vi "Funzioni stringhe.vi"() -> ()   [LabVIEW 2012]
panel:
  out "reversed":string
  out "first char last":string
  out "string array all'indice":string
  out "selection":bool
  out "match":string
  out "match + rest of string":string
  out "substring before match":string
  out "appended array":dbl[][](array[numeric])
  out "array":dbl[][](array[numeric])
  out "spreadsheet string":string
  out "number of replacements":i32
  out "result string dopo search e replace":string
  out "replaced substring":string
  out "result string dopo replace":string
  in  "Substringa":string="Pappappero"
  out "substring":string
  out "concatenated string":string
  out "length":i32
  in  "Stringa iniziale":string="Si sta come d'autunno sugli alberi le foglie."
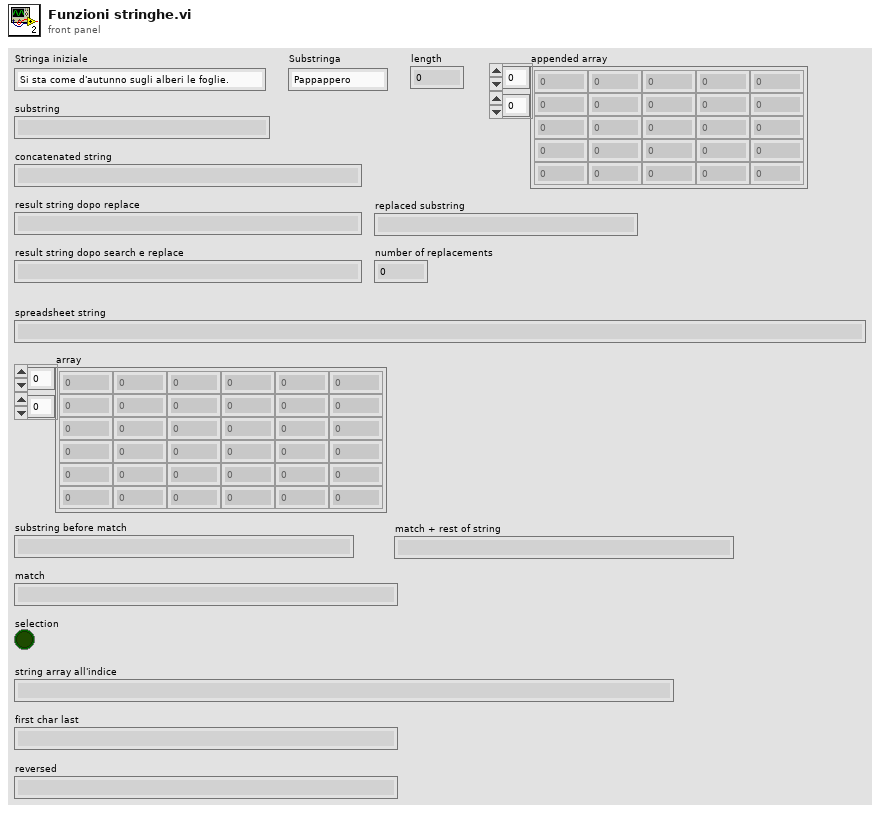
[diagram p1: front panel]
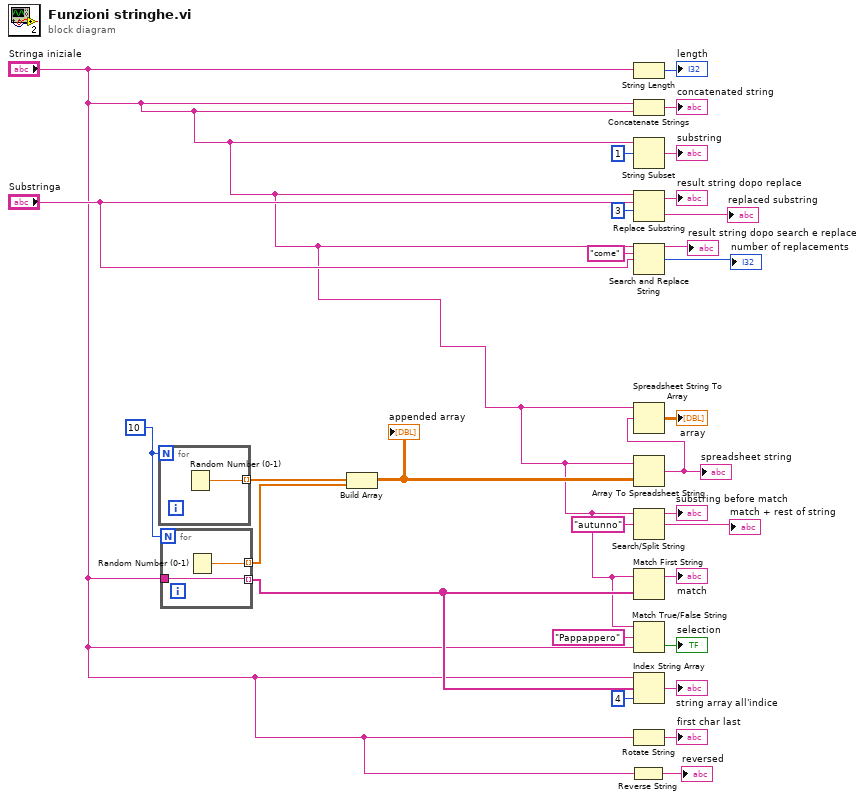
[diagram p0: block diagram]
diagram:
  w16 = 10
  n1 = for {
    N: w16 -> [_]
    tunnel: [w30] -> w17 mode=indexing
    n2 = Random Number (0-1)() -> (number: 0 to 1=w30:dbl)
  }
  n3 = for {
    N: w16 -> [_]
    tunnel: [w32] -> w18 mode=indexing
    tunnel: [w31] -> w8 mode=indexing
    tunnel: "Stringa iniziale" -> [w31]
    n4 = Random Number (0-1)() -> (number: 0 to 1=w32:dbl)
  }
  n5 = Build Array(w17, w18) -> (w15:dbl[][])
  "appended array" <- w15
  n6 = Reverse String(1:"Stringa iniziale") -> (0:→"reversed":string)
  n7 = String Length(string="Stringa iniziale") -> (length=→"length":i32)
  n8 = Concatenate Strings("Stringa iniziale", "Stringa iniziale") -> (→"concatenated string":string)
  n9 = String Subset(string="Stringa iniziale", offset (0)=1) -> (substring=→"substring":string)  [unwired: 1 in]
  n10 = Replace Substring(3:3 ("offset (0)"), 4:"Substringa", 5:"Stringa iniziale") -> (0:→"replaced substring":string, 1:→"result string dopo replace":string)  [unwired: 1 in]
  n11 = Search and Replace String(input string="Stringa iniziale", search string="come", replace string="Substringa") -> (result string=→"result string dopo search e replace":string, number of replacements=→"number of replacements":i32)  [unwired: 5 in, 2 out]
  n12 = Array To Spreadsheet String(array=w15, 3:"Stringa iniziale") -> (spreadsheet string=w14:string)  [unwired: 1 in]
  "spreadsheet string" <- w14
  n13 = Spreadsheet String To Array(format string="Stringa iniziale", spreadsheet string=w14) -> (array=→"array":dbl[][])  [unwired: 2 in]
  n14 = Search/Split String(string="Stringa iniziale", search string/char (-)="autunno") -> (substring before match=→"substring before match":string, match + rest of string=→"match + rest of string":string)  [unwired: 1 in, 1 out]
  n15 = Match First String(2:w8, 3:"Stringa iniziale") -> (1:→"match":string)  [unwired: 1 out]
  n16 = Match True/False String(2:"Stringa iniziale", 3:"Pappappero" ("true string"), 4:"Stringa iniziale") -> (0:→"selection":bool)  [unwired: 1 out]
  n17 = Index String Array(1:4 ("index"), 2:w8, 3:"Stringa iniziale") -> (0:→"string array all'indice":string)
  n18 = Rotate String(1:"Stringa iniziale") -> (0:→"first char last":string)
